vi "testOPC.vi"() -> ()   [LabVIEW 2024]
uses:
  <vilib>/OPCUA/controls/NodeIds.ctl
  <vilib>/OPCUA/controls/NodeId.ctl
  <vilib>/OPCUA/client/Multiple Read UInt32.vi
  <vilib>/OPCUA/NI OPC UA Client.lvlib
panel:
  in  "Stop Button":bool
  out "CounterOPC":u32
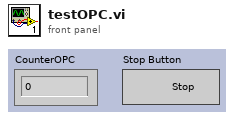
[diagram p1: front panel]
types:
  T1 = typedef "NodeIds.ctl" = T2[]
  T2 = typedef "NodeId.ctl" = string
  T3 = typedef "OPC UA Client Refnum.ctl" = refnum<k21>
  T4 = typedef "OPC UA StatusCode.ctl" = u32
  T5 = cluster{"node ID":T2, "value ":u32, "timestamp":timestamp, "status":T4}[]
  T6 = cluster{"node ID":T2, "value ":u32, "timestamp":timestamp, "status":T4}
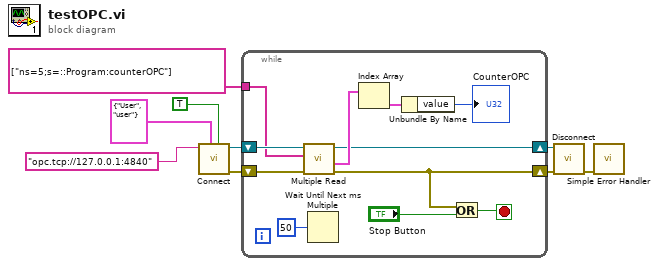
[diagram p0: block diagram]
diagram:
  n1 = call <vilib>:"Connect.vi"("trust any server (F)"=TRUE, "username/password"=cluster{"username":string, "password":string} {"username"="User", "password"="user"}, "server endpoint URL"="opc.tcp://127.0.0.1:4840") -> ("error out"=w2:errorcluster, "OPC UA client refnum out"=w5:T3)  [unwired: 6 in, 1 out]
  n2 = while {
    shift-right: [w15] -> w4
    shift-left: w5 -> [w19]
    tunnel: T1 ["ns=5;s=::Program:counterOPC"] ("node IDs") -> [w16]
    shift-right: [w11] -> w1
    shift-left: w2 -> [w14]
    stop <- w12 stop-if-true
    n3 = call-poly <vilib>:"Multiple Read.vi"("error in (no error)"=w14, "node IDs"=w16, "OPC UA client refnum in"=w19) -> ("error out"=w11:errorcluster, "results"=w18:T5, "OPC UA client refnum out"=w15:T3)  [unwired: 5 in, 1 out]
    n4 = Wait Until Next ms Multiple(millisecond multiple=u32 50) -> ()  [unwired: 1 out]
    n5 = Index Array(array=w18) -> (element=w17:T6)  [unwired: 1 in]
    n6 = Unbundle By Name(w17) -> ("value"=→"CounterOPC":u32)
    n7 = Or(x=w11, y="Stop Button") -> (x .or. y?=w12:bool)
  }
  n8 = call <vilib>:"Disconnect.vi"("error in (no error)"=w1, "OPC UA client refnum in"=w4) -> ("error out"=w9:errorcluster)  [unwired: 9 in]
  n9 = call <vilib>:"Simple Error Handler.vi"("error in (no error)"=w9) -> ()  [unwired: 4 in, 5 out]
